vi "test temp.vi"() -> ()   [LabVIEW 2018]
uses:
  <vilib>/Utility/xml.llb/Read From XML File(string).vi
panel:
  out "Array":string[](array[string])
  in  "error in (no error)":errorcluster
  # "9215\n9220"
  # "9219\n9220\n9220\n9208\n9213\n9213"
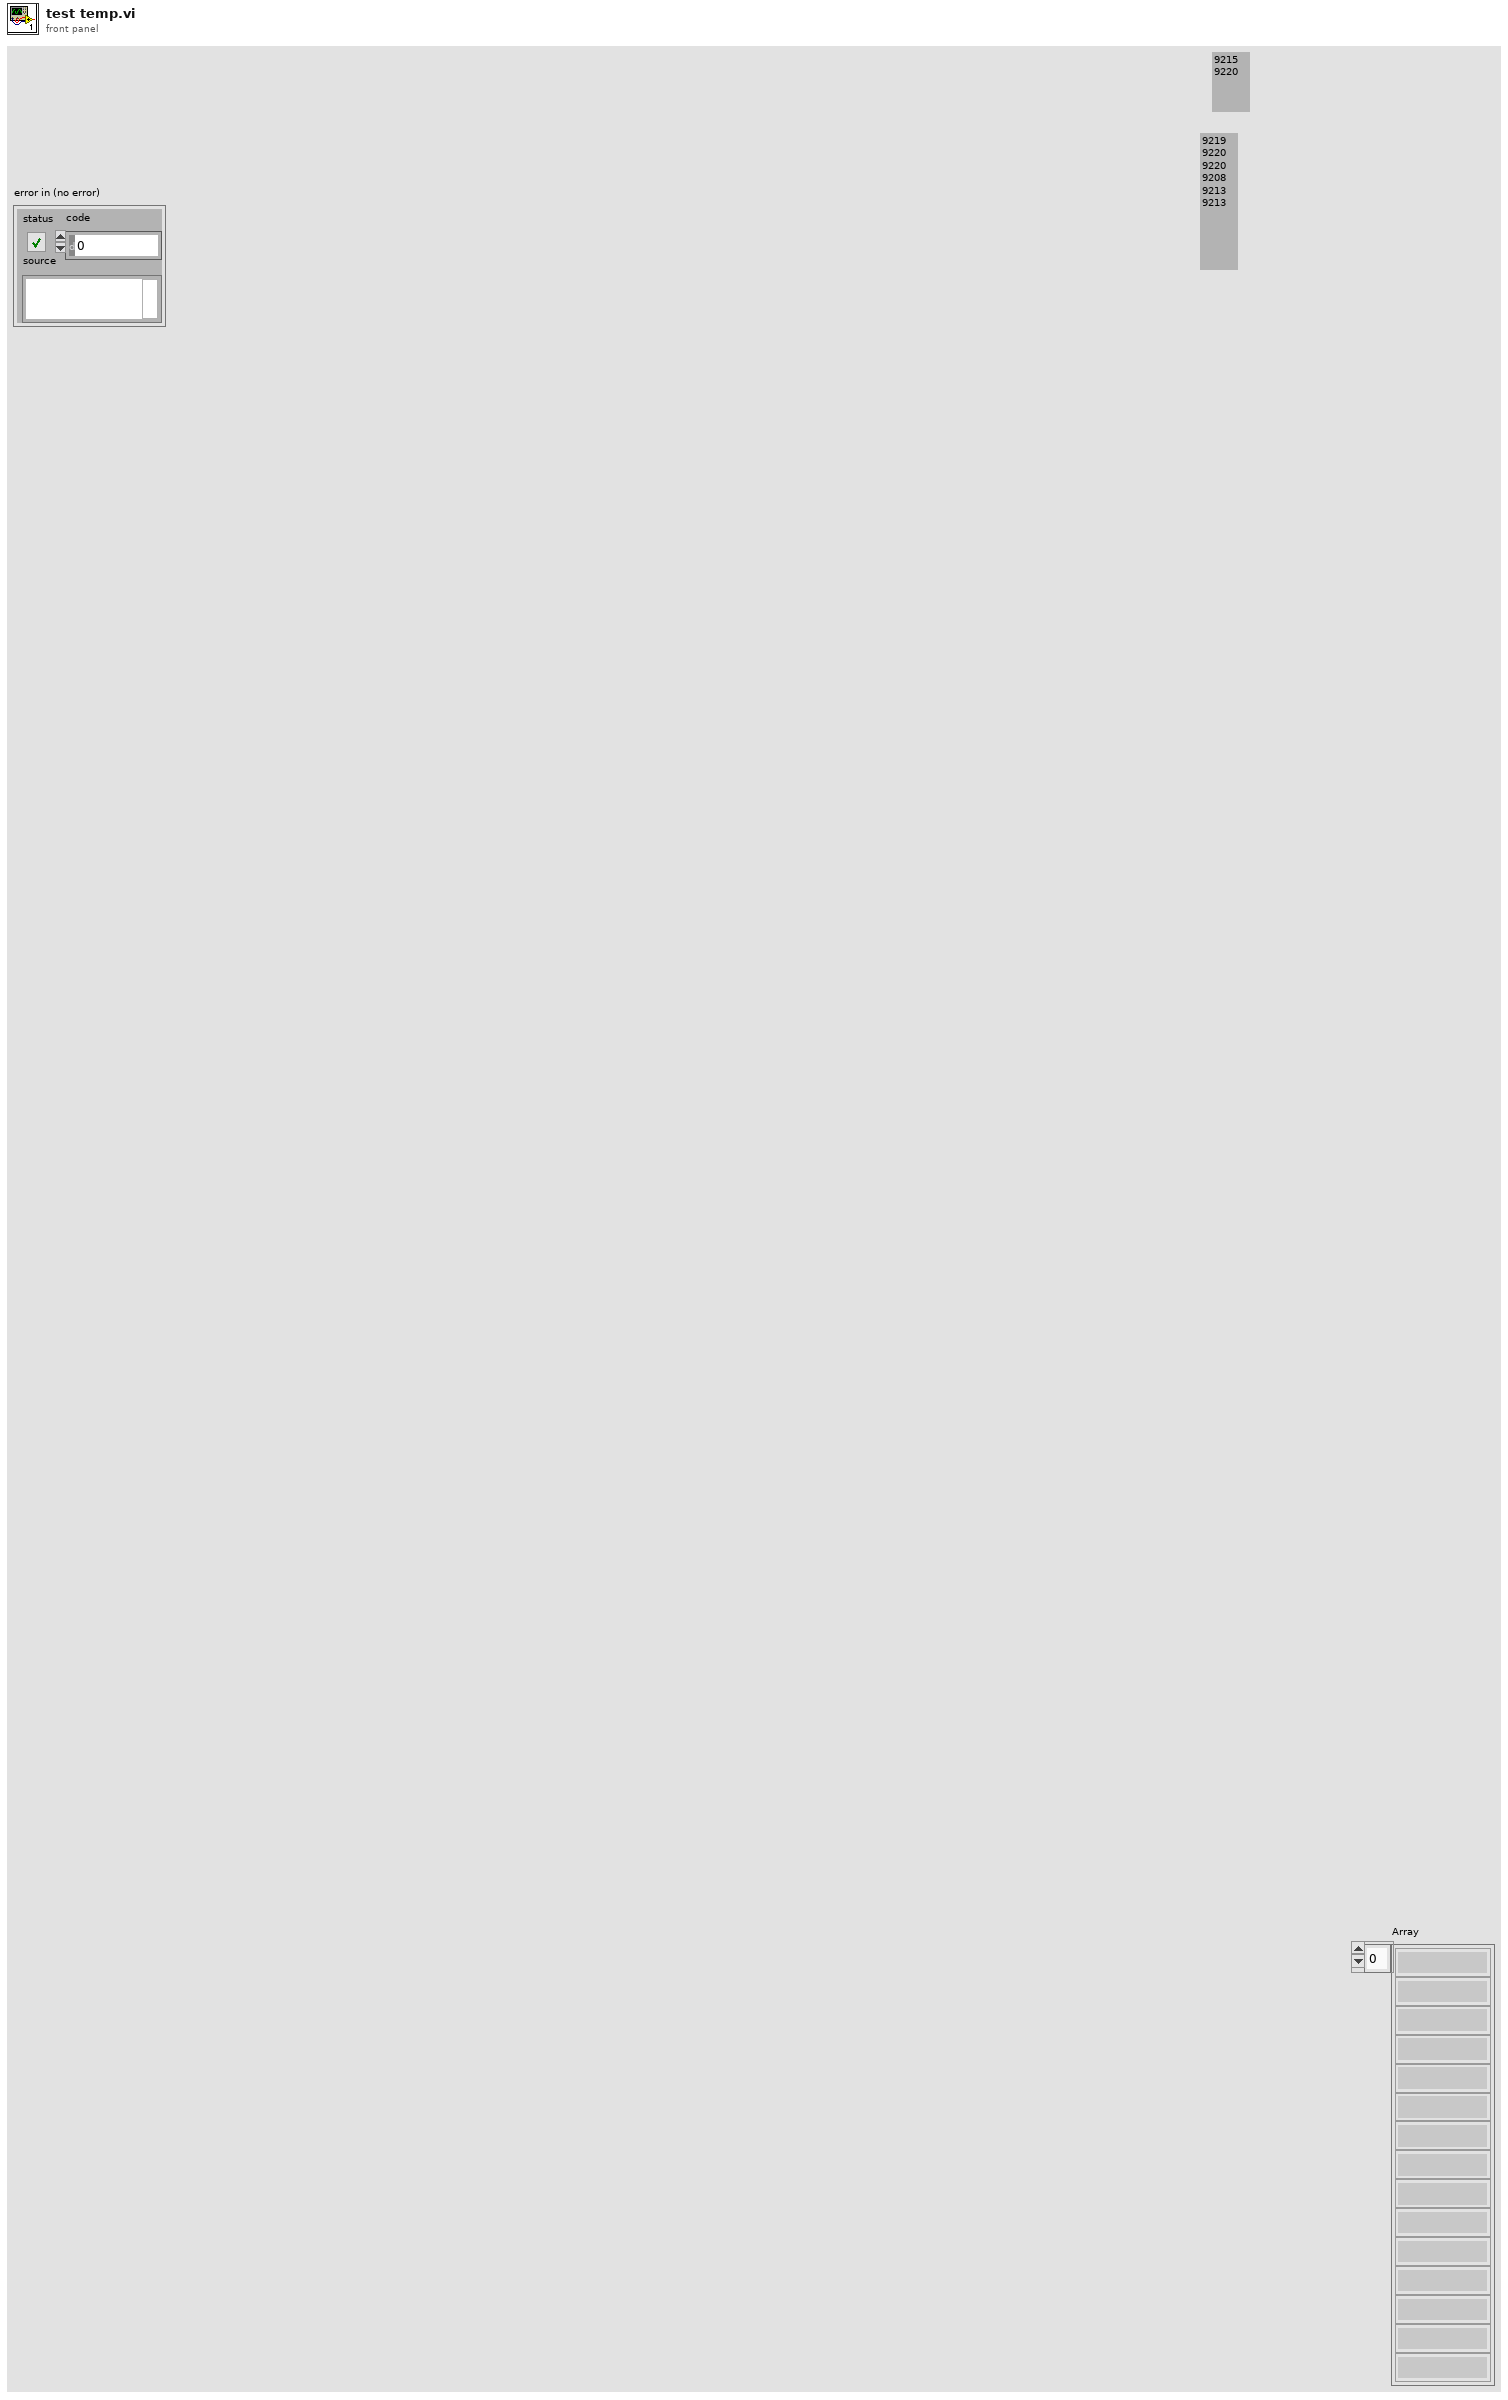
[diagram p1: front panel]
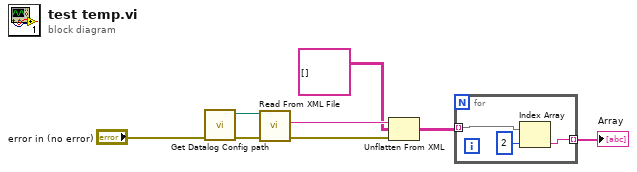
[diagram p0: block diagram]
diagram:
  n1 = call "Get Datalog Config path.vi"("error in (no error)"="error in (no error)") -> ("error out"=w4:errorcluster, "Data Log Config"=w5:path)  [unwired: 9 in]
  n2 = call-poly <vilib>:"Read From XML File.vi"("error in (no error)"=w4, "XML File Path"=w5) -> ("error out"=w7:errorcluster, "XML Elements"=w8:string)  [unwired: 7 in, 1 out]
  n3 = Unflatten From XML(xml string=w8, type=string[][] [], error in (no error)=w7) -> (value=w2:string[][])  [unwired: 1 out]
  n4 = for {
    tunnel: w2 -> [w10] mode=indexing
    tunnel: [w9] -> w1 mode=indexing
    n5 = Index Array(array=w10, index=2) -> (element=w9:string)
  }
  "Array" <- w1
